vi "buildPieceArray.vi"(8 "error in (no error)":errorcluster, 9 "Row":i32, 10 "Row":string, 11 "object in":refnum<class "Board.lvclass">) -> (0 "error out":errorcluster, 2 "Piece array":refnum<class "Piece.lvclass">[](array[class]), 3 "object out":refnum<class "Board.lvclass">)   [LabVIEW 2020, in "Board.lvclass"]
uses:
  Board.lvclass
  Pieces/Piece.lvclass
  Pieces/Queen/Queen.lvclass
  C:/_repos/_personal/Chess/Chess_LV/source/Pieces/Piece.lvclass
  Pieces/Rook/Rook.lvclass
  Pieces/Bishop/Bishop.lvclass
  Pieces/Knight/Knight.lvclass
  Pieces/Pawn/Pawn.lvclass
  Pieces/King/King.lvclass
  Board.lvclass/Board.ctl
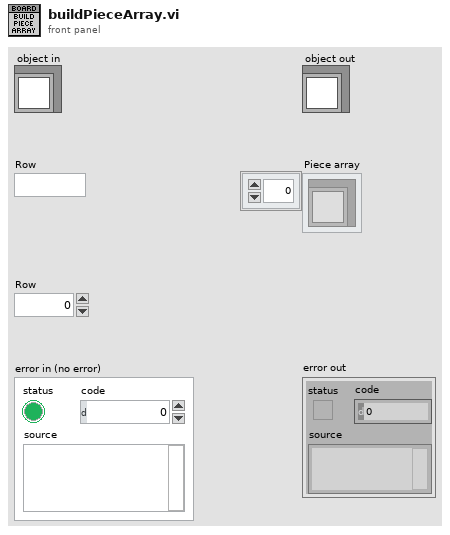
[diagram p1: front panel]
types:
  T1 = typedef "Piece.lvclass/pieceColor.ctl" = enum16{"white", "black"}
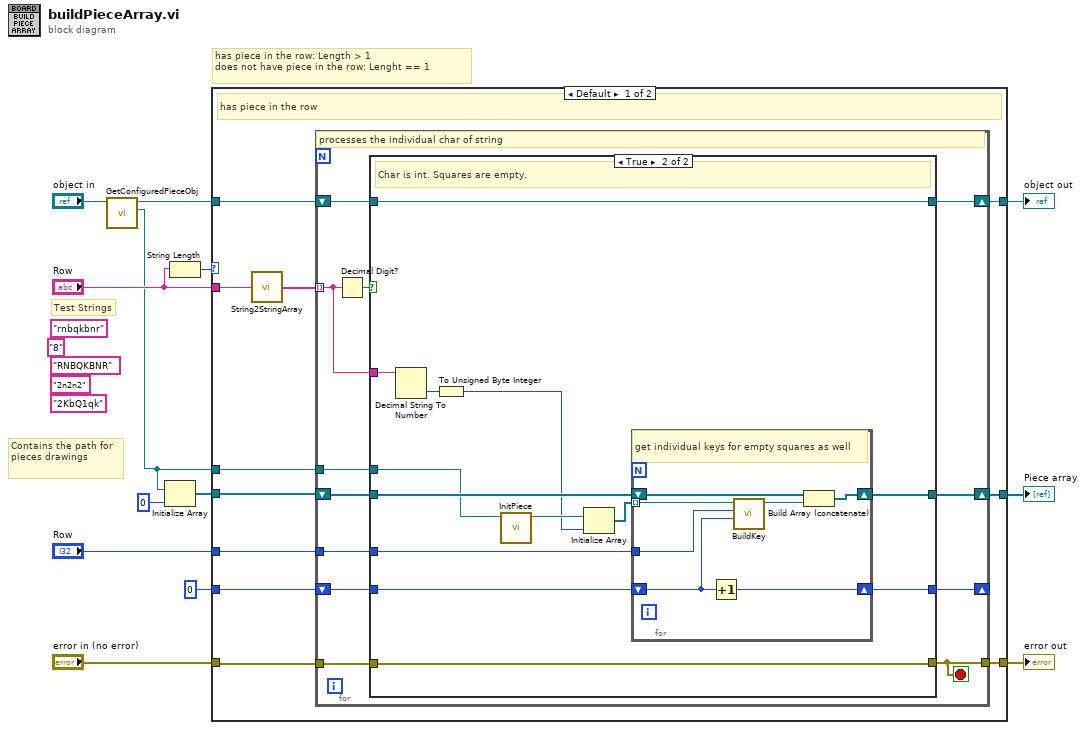
[diagram p0: block diagram]
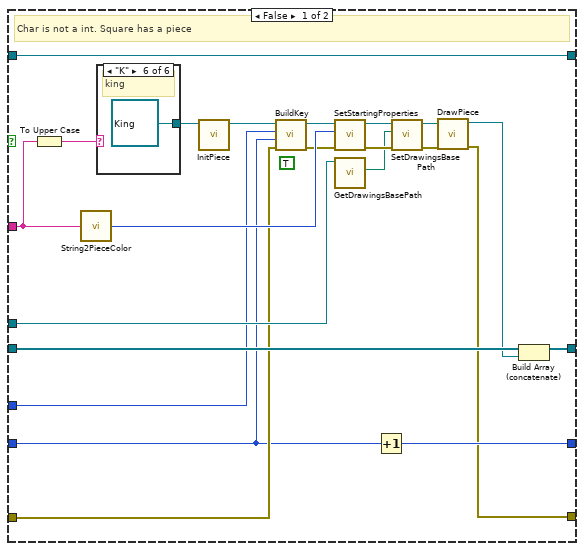
[diagram p2: hidden frame]
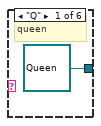
[diagram p3: hidden frame]
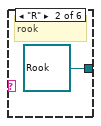
[diagram p4: hidden frame]
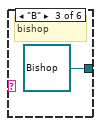
[diagram p5: hidden frame]
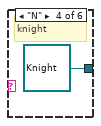
[diagram p6: hidden frame]
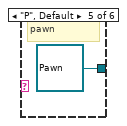
[diagram p7: hidden frame]
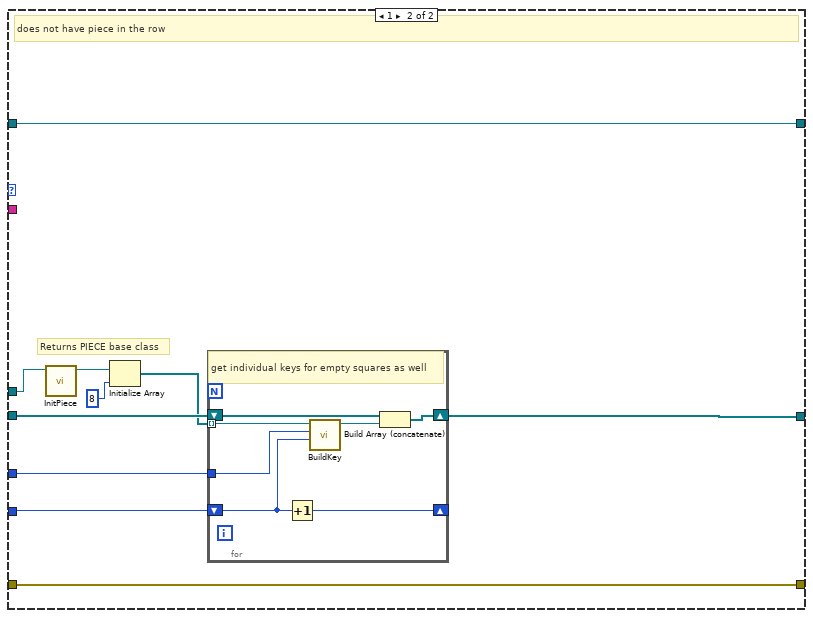
[diagram p8: hidden frame]
diagram:
  (unwired) "2KbQ1qk" ("token string")
  (unwired) "2n2n2" ("token string")
  (unwired) "RNBQKBNR" ("token string")
  (unwired) "8" ("token string")
  (unwired) "rnbqkbnr" ("token string")
  # "Contains the path for pieces drawings"
  # "Test Strings"
  # "has piece in the row: Length > 1\ndoes not have piece in the row: Lenght == 1"
  n1 = call "GetConfiguredPieceObj.vi"("object in"="object in") -> ("configuredPieceObj"=w1:refnum<class "Piece.lvclass">, "object out"=w2:refnum<class "Board.lvclass">)  [unwired: 8 in, 1 out]
  n2 = Initialize Array(w1, 0 ("dimension size")) -> (w6:refnum<class "Piece.lvclass">[])
  n3 = String Length(string="Row") -> (length=w13:i32)
  n4 = case shown="Default" w13 {
    tunnel: [w21 w88] -> w10
    tunnel: "Row" -> [w24 _]
    tunnel: w6 -> [w22 w93]
    tunnel: "Row" -> [w20 w87]
    tunnel: [w19 w92] -> w9
    tunnel: "error in (no error)" -> [w18 w92]
    tunnel: w1 -> [w17 w91]
    tunnel: 0 -> [w16 w86]
    tunnel: w2 -> [w15 w85]
    tunnel: [w14 w85] -> w3
    frame Default {
      # "has piece in the row"
      n5 = call "String2StringArray.vi"("String"=w24) -> ("Array of Char"=w23:string[])
      n6 = for {
        tunnel: w23 -> [w35] mode=indexing
        shift-right: [w33] -> w21
        shift-left: w22 -> [w34]
        shift-right: [w32] -> _
        shift-left: w16 -> [w31]
        tunnel: w20 -> [w30]
        tunnel: [w29] -> w19
        tunnel: w18 -> [w28]
        tunnel: w17 -> [w27]
        shift-right: [w25] -> w14
        shift-left: w15 -> [w26]
        stop <- w29 stop-if-true
        # "processes the individual char of string"
        n7 = Decimal Digit?(1:w35) -> (0:w36:bool)
        n8 = case shown="True" w36 {
          tunnel: w35 -> [w58 w77]
          tunnel: [w55 w75] -> w33
          tunnel: w34 -> [w56 w76]
          tunnel: [w54 w67] -> w32
          tunnel: w31 -> [w39 w66]
          tunnel: w30 -> [w40 w69]
          tunnel: [w52 w72] -> w29
          tunnel: w28 -> [w42 w72]
          tunnel: w27 -> [w46 w70]
          tunnel: w26 -> [w38 w65]
          tunnel: [w38 w65] -> w25
          frame False {
            (unwired) TRUE ("Init Game? (f)")
            # "Char is not a int. Square has a piece"
            n9 = To Upper Case(1:w58) -> (0:w57:string)
            n10 = call "String2PieceColor.vi"("String"=w58) -> ("Piece Color"=w45:T1)
            n11 = case shown="\"K\"" w57 {
              tunnel: [refnum<class "Queen.lvclass"> refnum ("Queen") refnum<class "Rook.lvclass"> refnum ("Rook") refnum<class "Bishop.lvclass"> refnum ("Bishop") refnum<class "Knight.lvclass"> refnum ("Knight") refnum<class "Pawn.lvclass"> refnum ("Pawn") refnum<class "King.lvclass"> refnum ("King")] -> w44
              frame "Q" {
                # "queen"
              }
              frame "R" {
                # "rook"
              }
              frame "B" {
                # "bishop"
              }
              frame "N" {
                # "knight"
              }
              frame "P", Default {
                # "pawn"
              }
              frame "K" {
                # "king"
              }
            }
            n12 = call-dynamic "InitPiece.vi"("object in"=w44) -> ("object out"=w37:refnum<class "Piece.lvclass">)  [unwired: 9 in, 1 out]
            n13 = call "BuildKey.vi"("error in (no error)"=w42, "Column (65=A)"=w39, "Row (>=1)"=w40, "object in"=w37) -> ("error out"=w41:errorcluster, "object out"=w43:refnum<class "Piece.lvclass">)  [unwired: 5 in, 1 out]
            n14 = call "SetStartingProperties.vi"("error in (no error)"=w41, "pieceColor"=w45, "object in"=w43) -> ("error out"=w51:errorcluster, "object out"=w49:refnum<class "Piece.lvclass">)  [unwired: 7 in]
            n15 = call "GetDrawingsBasePath.vi"("object in"=w46) -> ("drawingsBasePath"=w47:path)  [unwired: 8 in, 2 out]
            n16 = Increment(x=w39) -> (x+1=w54:i32)
            n17 = call "SetDrawingsBasePath.vi"("error in (no error)"=w51, "drawingsBasePath"=w47, "object in"=w49) -> ("error out"=w50:errorcluster, "object out"=w48:refnum<class "Piece.lvclass">)  [unwired: 7 in]
            n18 = call "DrawPiece.vi"("error in (no error)"=w50, "object in"=w48) -> ("error out"=w52:errorcluster, "object out"=w53:refnum<class "Piece.lvclass">)  [unwired: 8 in]
            n19 = Build Array (concatenate)(w56, w53) -> (w55:refnum<class "Piece.lvclass">[])
          }
          frame True {
            # "Char is int. Squares are empty."
            n20 = Decimal String To Number(string=w77) -> (number=w73:i32)  [unwired: 2 in, 1 out]
            n21 = To Unsigned Byte Integer(number=w73) -> (unsigned 8bit integer=w68:u8)
            n22 = call-dynamic "InitPiece.vi"("object in"=w70) -> ("object out"=w71:refnum<class "Piece.lvclass">)  [unwired: 9 in, 1 out]
            n23 = Initialize Array(w71, w68) -> (w74:refnum<class "Piece.lvclass">[])
            n24 = for {
              tunnel: w74 -> [w82] mode=indexing
              tunnel: w69 -> [w80]
              shift-right: [w79] -> w67
              shift-left: w66 -> [w78]
              shift-right: [w83] -> w75
              shift-left: w76 -> [w84]
              # "get individual keys for empty squares as well"
              n25 = Increment(x=w78) -> (x+1=w79:i32)
              n26 = call "BuildKey.vi"("Column (65=A)"=w78, "Row (>=1)"=w80, "object in"=w82) -> ("object out"=w81:refnum<class "Piece.lvclass">)  [unwired: 6 in, 2 out]
              n27 = Build Array (concatenate)(w84, w81) -> (w83:refnum<class "Piece.lvclass">[])
            }
          }
        }
      }
    }
    frame 1 {
      # "Returns PIECE base class"
      # "does not have piece in the row"
      n28 = call-dynamic "InitPiece.vi"("object in"=w91) -> ("object out"=w90:refnum<class "Piece.lvclass">)  [unwired: 9 in, 1 out]
      n29 = Initialize Array(w90, 8 ("dimension size")) -> (w89:refnum<class "Piece.lvclass">[])
      n30 = for {
        tunnel: w89 -> [w99] mode=indexing
        tunnel: w87 -> [w97]
        shift-right: [w96] -> _
        shift-left: w86 -> [w95]
        shift-right: [w100] -> w88
        shift-left: w93 -> [w101]
        # "get individual keys for empty squares as well"
        n31 = Increment(x=w95) -> (x+1=w96:i32)
        n32 = call "BuildKey.vi"("Column (65=A)"=w95, "Row (>=1)"=w97, "object in"=w99) -> ("object out"=w98:refnum<class "Piece.lvclass">)  [unwired: 6 in, 2 out]
        n33 = Build Array (concatenate)(w101, w98) -> (w100:refnum<class "Piece.lvclass">[])
      }
    }
  }
  "Piece array" <- w10
  "error out" <- w9
  "object out" <- w3
